vi "serial_AUCT_comp_p4.vi"() -> ()   [LabVIEW 2018]
uses:
  Controls created/Control 3.ctl
  Controls created/Control 4.ctl
  <vilib>/Instr/_visa.llb/VISA Configure Serial Port (Instr).vi
  <instrlib>/LeCroy Wave Series/Public/Data/Read Single Waveform.vi
  <vilib>/Utility/file.llb/Read Delimited Spreadsheet (DBL).vi
  <vilib>/Utility/file.llb/Write Delimited Spreadsheet (DBL).vi
  <instrlib>/Siglent SDG X Series/Siglent SDG X Series.lvlib
  <instrlib>/LeCroy Wave Series/LeCroy Wave Series.lvlib
panel:
  out "relative seconds 2":dbl format="%_19f"
  out "relative seconds":dbl
  out "Array":dbl[][](array[numeric])
  in  "Tab Control":T1(tab)
  in  "Scanning Distance(in mm)":i32=26
  in  "Experiment Dir":path=path "E:/Ankur/Labview/Automation/Data"
  in  "Exp_name":string="Test1"
  out "Exp_dir out dir":path
  out "Proc_data out dir":path
  out "Dis_step":dbl
  in  "Trend":dbl
  in  "N_packets":dbl=7.0
  out "Sinogram":dbl[][](graph)
  out "Reconstruction":dbl[][](graph)
  in  "VISA resource":refnum<visa-resource-name>="COM5"
  in  "NR":i16=10
  in  "Set Speed (Steps/s)":i16=900 min=0 max=3000 step=50
  in  "Baud Rate":u32=9600
  out "Iteration #":i32
  in  "NT":i16=10
  out "Error":errorcluster
  in  "Arbitray Movement":bool
  out "stop motion":bool
  in  "MOTION":bool
  in  "?":i8(slide) step=2 scale=0.0..2.0
  in  "OK Button":bool
  out "# NT":i32
  in  "ms to wait(Translation)":u32=100
  in  "milliseconds to wait":u32=100
  in  "ms to wait(Rotation)":u32=100
  out "Code Part Time":dbl[](array[numeric])
  out "gr_time":dbl
  in  "VISA Refnum in":refnum<visa-resource-name>="USB0::0xF4EC::0xEE38::SDG2XCAD2R3765::INSTR"
  in  "Channel (1:Channel 1)":i32(ring)=1 items=["Channel 1"=1, "Channel 2"=2]
  in  "Enable Output (T: Enable)":bool=TRUE
  in  "Amplitude (1.0 Vpp)":dbl=20.0 format="%#.3f"
  in  "Frequency (1000 Hz)":T2=1500000.0 format="%#.6g"
  in  "DC Offset (0.00 V) in":dbl
  in  "Waveform Function (0: Sine) in":u16(ring) items=["Sine", "Square", "Ramp", "DC", "Pulse", "Arb"]
  in  "Phase (0.0 degrees)":dbl=0.002 min=-360.0 max=360.0 format="%#.1g"
  in  "Fall (20 ns)":dbl=8.4e-09 format="%#.3g"
  in  "Duty (20%)":dbl=4.32 min=0.0001 max=100.0 format="%.4g"
  in  "Delay (0.00 s)":dbl min=-1000000.0 max=1000000.0
  in  "Rise (20 ns)":dbl=1.04e-08 format="%#.3g"
  in  "True To \ngenerate\n pulse":T3=TRUE
  out "VISA resource name out":refnum<visa-resource-name>
  out "error out":errorcluster
  out "Output Filename":path
  out "error out 2":errorcluster
  in  "format string":string="Channel: %g \nWavetype: %g \nAMP: %gV\nFreq: %gHz \nRiseTime: %gs \nFallTime: %gs \nDutyCycle: %g"
  out "Oscilloscope\n Runnning":bool
  in  "stop":bool
  out "Waveform Data":waveform(dbl)(graph)
  in  "Source (0: Channel 1)":u16(ring) items=["Channel 1", "Channel 2", "Channel 3", "Channel 4", "Memory 1", "Memory 2", "Memory 3", "Memory 4", "Function 1", "Function 2", "Function 3", "Function 4", "Function 5", "Function 6", "Function 7", "Function 8"]
  in  "Perform Auto Setup?":bool
  in  "Save Files in Directory (In Oscilloscope)":string="D:\\Automation\\Data"
  in  "Filename":string="Title"
  out "Saved filename":string
  out "Error Dsocom":errorcluster
  in  "VISA resource name":refnum<visa-resource-name>="USB0::0x05FF::0x1023::3517N53447::INSTR"
  in  "Reset Scope?":bool
  out "VISA DSO":refnum<visa-resource-name>
  # "For Rotational motion"
  # "For Translational Motion"
  # "For Translational motion"
  # "OFF"
  # "ON"
  # "Instr conn"
  # "Scan. loop"
  # "All Comb"
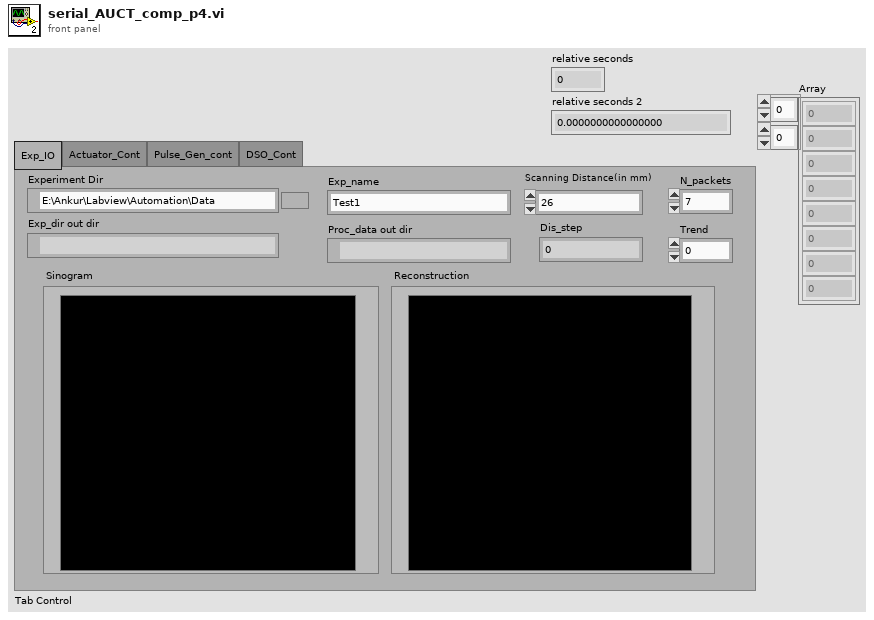
[diagram p1: front panel]
types:
  T1 = enum32{"Exp_IO", "Actuator_Cont", "Pulse_Gen_cont", "DSO_Cont"}
  T2 = typedef "Control 3.ctl" = dbl
  T3 = typedef "Control 4.ctl" = bool
  T4 = enum16{"open", "replace", "create", "open or create", "replace or create", "replace or create with confirmation"}
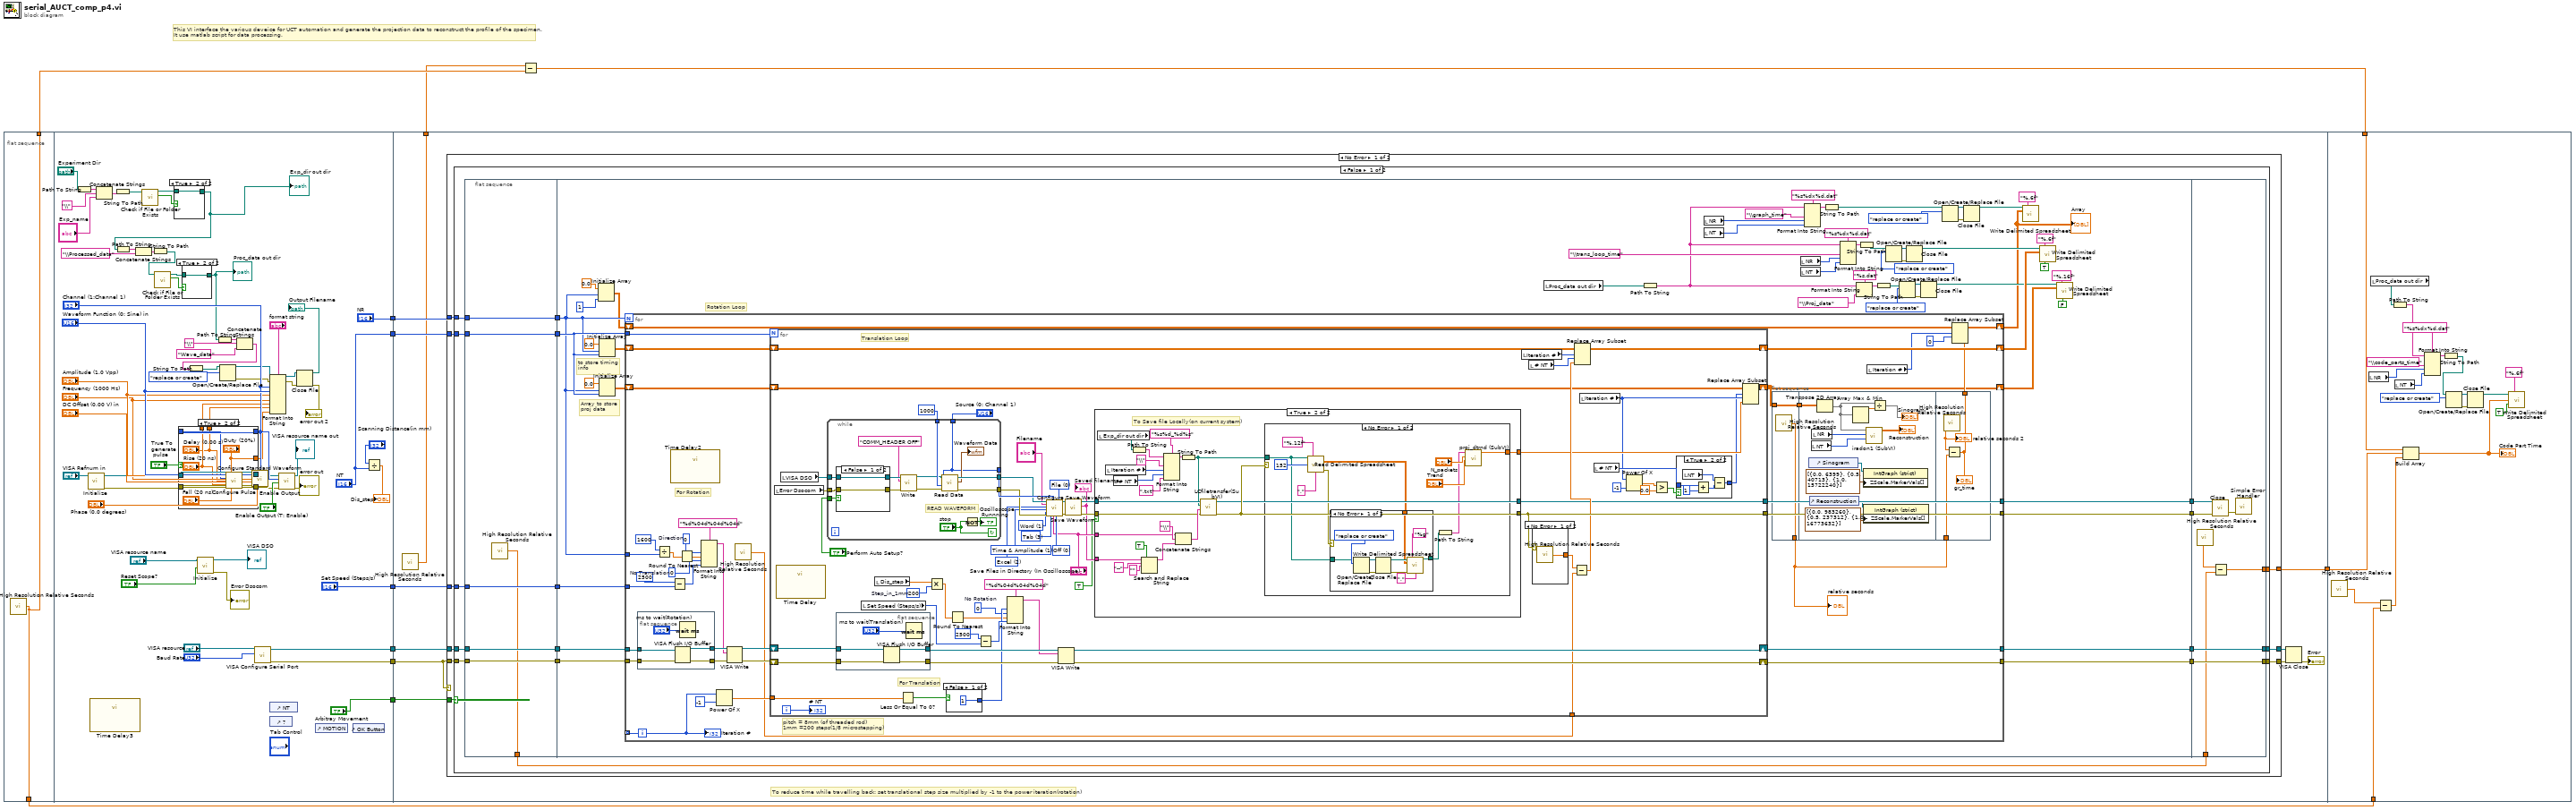
[diagram p0: block diagram]
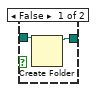
[diagram p2: hidden frame]
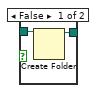
[diagram p3: hidden frame]
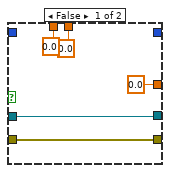
[diagram p4: hidden frame]
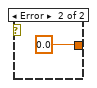
[diagram p6: hidden frame]
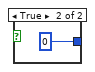
[diagram p7: hidden frame]
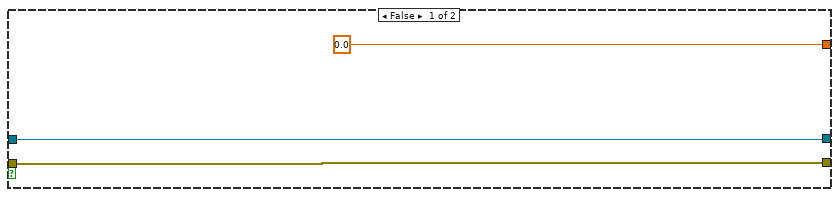
[diagram p8: hidden frame]
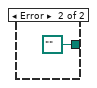
[diagram p9: hidden frame]
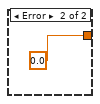
[diagram p10: hidden frame]
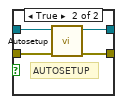
[diagram p11: hidden frame]
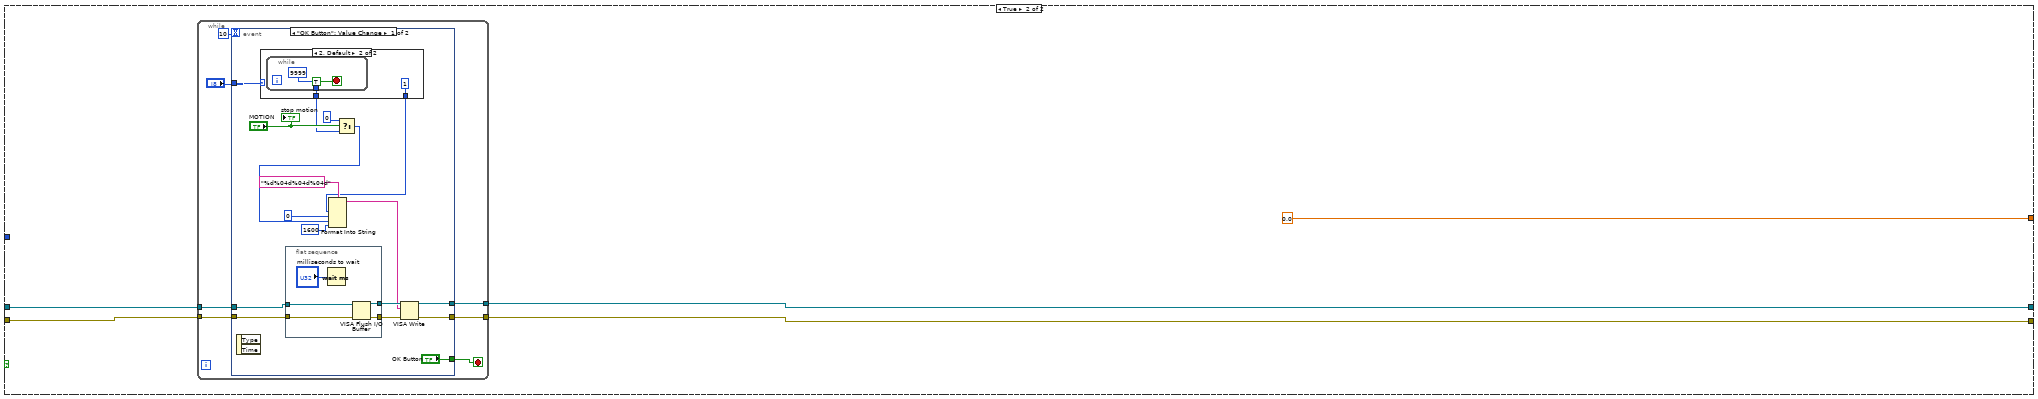
[diagram p12: hidden frame]
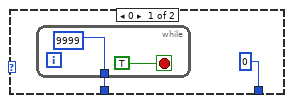
[diagram p13: hidden frame]
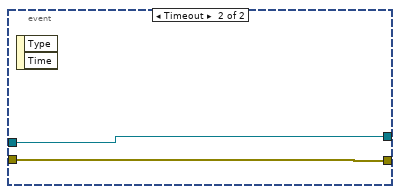
[diagram p14: hidden frame]
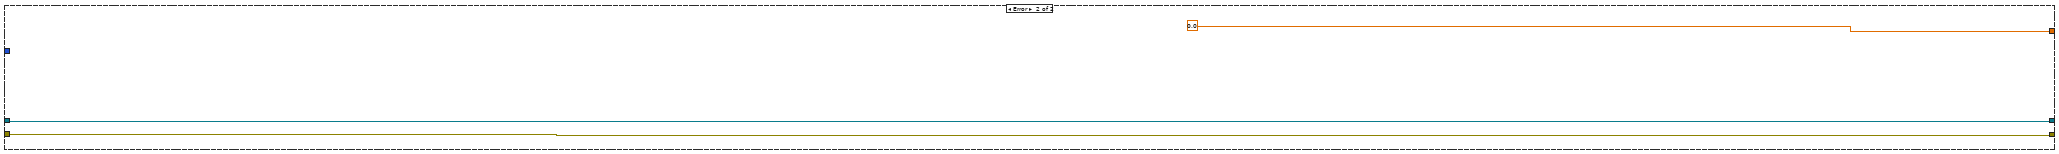
[diagram p15: hidden frame]
diagram:
  # "This VI interface the various deveice for UCT automation and generate the projection data to reconstruct the profile of the specimen.\nIt use matlab script for data processing."
  n1 = flat-sequence {
    tunnel: [w12] -> w3
    tunnel: [w12] -> w2
    tunnel: ["NT"] -> w11
    tunnel: [w41] -> w10
    tunnel: [w40] -> w9
    tunnel: ["Arbitray Movement"] -> w8
    tunnel: ["Set Speed (Steps/s)"] -> w7
    tunnel: ["NR"] -> w6
    tunnel: w11 -> [w103]
    tunnel: w10 -> [w102]
    tunnel: w9 -> [w101]
    tunnel: w8 -> [w100]
    tunnel: w7 -> [w99]
    tunnel: w6 -> [w98]
    tunnel: [w97] -> w4
    tunnel: [w96] -> w1
    tunnel: w5 -> [w471]
    tunnel: w4 -> [w470]
    tunnel: w3 -> [w469]
    frame #0 {
      n2 = call <vilib>:"High Resolution Relative Seconds.vi"() -> ("relative seconds"=w12:dbl)
    }
    frame #1 {
      n3 = Path To String(path="Experiment Dir") -> (string=w34:string)
      n4 = call <instrlib>:"Initialize.vi"("VISA resource name"="VISA Refnum in") -> ("error out"=w48:errorcluster, "VISA resource name out"=w47:refnum<visa-resource-name>)  [unwired: 9 in]
      n5 = call "Time Delay3"() -> ()  [unwired: 11 in, 1 out]
      n6 = Concatenate Strings(w34, "\\" ("string"), "Exp_name") -> (w32:string)
      n7 = String To Path(string=w32) -> (path=w28:path)
      n8 = call <vilib>:"Check if File or Folder Exists.vi"("path"=w28) -> ("file or folder exists?"=w27:bool, "dup path"=w26:path)  [unwired: 8 in, 1 out]
      n9 = case shown="True" w27 {
        tunnel: w26 -> [w80 w81]
        tunnel: [w79 w81] -> w22
        frame False {
          n10 = Create Folder(path (use dialog)=w80) -> (created path=w79:path)  [unwired: 2 in, 2 out]
        }
        frame True {
        }
      }
      "Exp_dir out dir" <- w22
      n11 = Path To String(path=w22) -> (string=w36:string)
      n12 = Concatenate Strings(w36, "\\Processed_data" ("string")) -> (w35:string)
      n13 = String To Path(string=w35) -> (path=w23:path)
      n14 = call <vilib>:"Check if File or Folder Exists.vi"("path"=w23) -> ("file or folder exists?"=w25:bool, "dup path"=w24:path)  [unwired: 8 in, 1 out]
      n15 = case shown="True" w25 {
        tunnel: [w77 w78] -> w19
        tunnel: w24 -> [w76 w78]
        frame False {
          n16 = Create Folder(path (use dialog)=w76) -> (created path=w77:path)  [unwired: 2 in, 2 out]
        }
        frame True {
        }
      }
      "Proc_data out dir" <- w19
      n17 = call <instrlib>:"Initialize.vi"("Reset? (T: Yes)"="Reset Scope?", "VISA resource name"="VISA resource name") -> ("error out"=→"Error Dsocom":errorcluster, "VISA resource name out"=→"VISA DSO":refnum<visa-resource-name>)  [unwired: 8 in]
      n18 = Path To String(path=w19) -> (string=w20:string)
      n19 = Concatenate Strings(w20, "\\" ("string"), "Wave_data" ("Filename")) -> (w16:string)
      n20 = String To Path(string=w16) -> (path=w15:path)
      n21 = Open/Create/Replace File(file path (use dialog)=w15, operation (0:open)=T4."replace or create") -> (refnum out=w21:refnum<file>, error out=w13:errorcluster)  [unwired: 4 in, 1 out]
      n22 = call <instrlib>:"Configure Standard Waveform.vi"("VISA resource name"=w47, "Waveform Function (0: Sine)"="Waveform Function (0: Sine) in", "Channel (1:Channel 1)"="Channel (1:Channel 1)", "Amplitude (1.0 Vpp)"="Amplitude (1.0 Vpp)", "Frequency (1000 Hz)"="Frequency (1000 Hz)", "DC Offset (0.00 V)"="DC Offset (0.00 V) in", "error in (no error)"=w48, "Phase (0.0 degrees)"="Phase (0.0 degrees)") -> ("VISA resource name out"=w52:refnum<visa-resource-name>, "error out"=w49:errorcluster)  [unwired: 6 in]
      n23 = case shown="True" "True To \ngenerate\n pulse" {
        tunnel: [w86 w94] -> w43
        tunnel: [w85 w93] -> w44
        tunnel: w52 -> [w86 w92]
        tunnel: w49 -> [w85 w91]
        tunnel: "Channel (1:Channel 1)" -> [_ w90]
        tunnel: "Channel (1:Channel 1)" -> [_ _]
        tunnel: [0.0 ("Duty (20%)") "Duty (20%)"] -> w56
        tunnel: [0.0 ("Rise (20 ns)") "Rise (20 ns)"] -> w64
        tunnel: [0.0 ("Delay (0.00 s)") "Delay (0.00 s)"] -> w65
        frame False {
        }
        frame True {
          n24 = call <instrlib>:"Configure Pulse.vi"("VISA resource name"=w92, "Duty (20%)"="Duty (20%)", "Channel (1:Channel 1)"=w90, "Delay (0.00 s)"="Delay (0.00 s)", "Rise (20 ns)"="Rise (20 ns)", "error in (no error)"=w91, "Fall (20 ns)"="Fall (20 ns)") -> ("VISA resource name out"=w94:refnum<visa-resource-name>, "error out"=w93:errorcluster)  [unwired: 7 in]
        }
      }
      n25 = call-poly "VISA Configure Serial Port"("VISA resource name"="VISA resource", "baud rate (9600)"="Baud Rate") -> ("VISA resource name out"=w41:refnum<visa-resource-name>, "error out"=w40:errorcluster)  [unwired: 12 in]
      n26 = Format Into String(format string="format string", initial string=w21, error in=w13, "Channel (1:Channel 1)", "Waveform Function (0: Sine) in", "Amplitude (1.0 Vpp)", "Frequency (1000 Hz)", w64, w65, w56) -> (resulting string=w57:refnum<file>, error out=w60:errorcluster)
      n27 = control-ref of="NT"() -> ()  [unwired: 1 out]
      n28 = control-ref of="?"() -> ()  [unwired: 1 out]
      n29 = call <instrlib>:"Enable Output.vi"("error in (no error)"=w44, "Enable Output (T: Enable)"="Enable Output (T: Enable)", "Channel (1:Channel 1)"="Channel (1:Channel 1)", "VISA resource name"=w43) -> ("error out"=→"error out":errorcluster, "VISA resource name out"=→"VISA resource name out":refnum<visa-resource-name>)  [unwired: 6 in]
      n30 = Close File(refnum=w57, error in=w60) -> (path=→"Output Filename":path, error out=→"error out 2":errorcluster)
      n31 = control-ref of="MOTION"() -> ()  [unwired: 1 out]
      n32 = control-ref of="OK Button"() -> ()  [unwired: 1 out]
      n33 = Divide(x="Scanning Distance(in mm)", y="NT") -> (x/y=→"Dis_step":dbl)
    }
    frame #2 {
      # "To reduce time while travelling back: set translational step size multiplied by -1 to the power iteration(rotation)"
      n34 = call <vilib>:"High Resolution Relative Seconds.vi"() -> ("relative seconds"=w96:dbl)
      n35 = case shown="No Error" w101 {
        tunnel: [w108 w451] -> w106
        tunnel: w98 -> [w115 _]
        tunnel: w99 -> [w114 _]
        tunnel: w100 -> [w113 _]
        tunnel: w101 -> [w112 w451]
        tunnel: w102 -> [w111 w450]
        tunnel: w103 -> [w110 _]
        tunnel: [w109 w450] -> w104
        tunnel: [w107 0.0] -> w97
        frame No Error {
          n36 = case shown="False" w113 {
            tunnel: w115 -> [w130 _]
            tunnel: w114 -> [w133 _]
            tunnel: w112 -> [w132 w409]
            tunnel: w111 -> [w131 w408]
            tunnel: w110 -> [w129 _]
            tunnel: [w128 w407] -> w109
            tunnel: [w118 w406] -> w108
            tunnel: [w117 0.0] -> w107
            frame False {
              n37 = flat-sequence {
                tunnel: w129 -> [w135]
                tunnel: w130 -> [w136]
                tunnel: w131 -> [w137]
                tunnel: w132 -> [w138]
                tunnel: w133 -> [w139]
                tunnel: [w139] -> w125
                tunnel: [w138] -> w124
                tunnel: [w137] -> w123
                tunnel: [w136] -> w122
                tunnel: [w135] -> w121
                tunnel: [w134] -> w116
                tunnel: [w190] -> w127
                tunnel: [w189] -> w126
                tunnel: w125 -> [w193]
                tunnel: w124 -> [w192]
                tunnel: w123 -> [w191]
                tunnel: w122 -> [w143]
                tunnel: w121 -> [w170]
                tunnel: [w188] -> w120
                tunnel: [w187] -> w119
                tunnel: [w404] -> w128
                tunnel: w127 -> [w404]
                tunnel: w126 -> [w400]
                tunnel: w120 -> [w402]
                tunnel: w119 -> [w401]
                tunnel: [w400] -> w118
                tunnel: [w398] -> w117
                tunnel: w116 -> [w397]
                frame #0 {
                  n38 = call <vilib>:"High Resolution Relative Seconds.vi"() -> ("relative seconds"=w134:dbl)
                }
                frame #1 {
                  # "to store timing\ninfo"
                  # "Array to store \nproj data"
                  # "Rotation Loop"
                  n39 = Initialize Array(0.0 ("element"), w143, 1 ("dimension size")) -> (w142:dbl[][])
                  n40 = Initialize Array(0.0, w143, w170) -> (w173:dbl[][])
                  n41 = Initialize Array(0.0, w143, w170) -> (w169:dbl[][])
                  n42 = for {
                    N: w143 -> [_]
                    tunnel: [w227] -> w189
                    tunnel: [w228] -> w190
                    tunnel: w193 -> [w208]
                    tunnel: [w230] -> _ mode=indexing
                    tunnel: w192 -> [w221]
                    tunnel: w191 -> [w222]
                    tunnel: w143 -> [w214]
                    tunnel: w170 -> [w210]
                    tunnel: [w207] -> w188
                    tunnel: [w206] -> w187
                    shift-right: [w203] -> w172
                    shift-left: w173 -> [w204]
                    shift-right: [w194] -> w157
                    shift-left: w169 -> [w202]
                    shift-right: [w199] -> w141
                    shift-left: w142 -> [w200]
                    i -> [w230]
                    w218 = 0  # No Translation
                    w216 = 0  # Direction
                    # "pitch = 8mm (of threaded rod)\n1mm =200 steps(1/8 microstepping)"
                    # "For Rotation"
                    n43 = flat-sequence {
                      tunnel: [w251] -> w225
                      tunnel: [w250] -> w226
                      tunnel: w222 -> [w248]
                      tunnel: w221 -> [w247]
                      frame #0 {
                        n44 = VISA Flush I/O Buffer(VISA resource name=w248, error in (no error)=w247) -> (VISA resource name out=w251:refnum<visa-resource-name>, error out=w250:errorcluster)  [unwired: 1 in]
                        n45 = Wait (ms)(milliseconds to wait="ms to wait(Rotation)") -> ()  [unwired: 1 out]
                      }
                    }
                    n46 = Divide(x=i16 1600, y=w214) -> (x/y=w213:dbl)
                    n47 = call "Time Delay2"() -> ()  [unwired: 11 in, 1 out]
                    n48 = Subtract(x=i16 2500 ("y"), y=w208) -> (x-y=w217:i16)
                    n49 = Round To Nearest(number=w213) -> (nearest integer value=w212:dbl)
                    n50 = Format Into String(format string="%d%04d%04d%04d", w216, w212, w218, w217) -> (resulting string=w220:string)  [unwired: 2 in, 1 out]
                    n51 = Power Of X(1:-1 ("x"), 2:w230) -> (0:w211:dbl)
                    n52 = VISA Write(VISA resource name=w225, write buffer=w220, error in (no error)=w226) -> (VISA resource name out=w223:refnum<visa-resource-name>, error out=w224:errorcluster)  [unwired: 1 out]
                    n53 = call <vilib>:"High Resolution Relative Seconds.vi"() -> ("relative seconds"=w205:dbl)
                    n54 = for {
                      N: w210 -> [_]
                      shift-right: [w281] -> w228
                      shift-left: w223 -> [w291]
                      shift-right: [w280] -> w227
                      shift-left: w224 -> [w290]
                      tunnel: w211 -> [w284]
                      tunnel: [w272] -> w207
                      tunnel: [w260] -> w206
                      tunnel: w205 -> [w270]
                      shift-right: [w268] -> w203
                      shift-left: w204 -> [w265]
                      shift-right: [w252] -> w194
                      shift-left: w202 -> [w264]
                      i -> [w312]
                      w276 = 200  # Step_in_1mm
                      w279 = 0  # No Rotation
                      w302 = u16 3 items=["Comma", "Space", "Semicolon", "Tab"] ("Delimiter (  0:Comma)")
                      w301 = u16 0 items=["Off", "Wrap", "Fill"] ("Auto Save (0:Off")
                      w303 = u16 1 items=["Byte", "Word", "Auto"] ("BinarySubFormat (1: Word)")
                      w304 = u16 1 items=["Amplitude Only", "Time & Amplitude", "With Header"] ("SubFormat (1: Time & Amplitude)")
                      w305 = u16 2 items=["Binary", "ASCII", "Excel", "MATLAB", "MathCad", "WaveML"] ("Format (0: Binary)")
                      w300 = u16 0 items=["File", "M1", "M2", "M3", "M4"] ("Destination (0:File)")
                      # "Translation Loop"
                      # "For Translation"
                      n55 = local read "Error Dsocom"() -> (w261:errorcluster)
                      n56 = call "Time Delay"() -> ()  [unwired: 11 in, 1 out]
                      n57 = local read "VISA DSO"() -> (w262:refnum<visa-resource-name>)
                      n58 = while {
                        tunnel: [w390] -> w310
                        tunnel: [w389] -> w309
                        tunnel: "Perform Auto Setup?" -> [w388]
                        tunnel: "Source (0: Channel 1)" -> [w382]
                        tunnel: w262 -> [w387]
                        tunnel: u32 1000 ("Timeout (10000 ms)") -> [w386]
                        tunnel: [w382] -> w311
                        tunnel: w261 -> [w381]
                        stop <- "stop" continue-if-true
                        # "READ WAVEFORM"
                        n59 = case shown="False" w388 {
                          tunnel: w381 -> [w391 w396]
                          tunnel: w387 -> [w392 w395]
                          tunnel: [w392 w394] -> w378
                          tunnel: [w391 w393] -> w377
                          frame False {
                          }
                          frame True {
                            # "AUTOSETUP"
                            n60 = call <instrlib>:"Autosetup.vi"("error in (no error)"=w396, "VISA resource name"=w395) -> ("error out"=w393:errorcluster, "VISA resource name out"=w394:refnum<visa-resource-name>)  [unwired: 8 in]
                          }
                        }
                        n61 = call <instrlib>:"Write.vi"("error in (no error)"=w377, "Write Buffer"="COMM_HEADER OFF", "VISA resource name"=w378) -> ("error out"=w379:errorcluster, "VISA resource name out"=w380:refnum<visa-resource-name>)  [unwired: 7 in]
                        n62 = call-poly <instrlib>:"Read Data.vi"("error in (no error)"=w379, "Timeout (10000 ms)"=w386, "Source (0: Channel 1)"=w382, "VISA resource name"=w380) -> ("error out"=w390:errorcluster, "Waveform Data"=→"Waveform Data":waveform(dbl), "VISA resource name out"=w389:refnum<visa-resource-name>)  [unwired: 5 in]
                        n63 = Not(x="stop") -> (.not. x?=→"Oscilloscope\n Runnning":bool)
                      }
                      n64 = flat-sequence {
                        tunnel: [w327] -> w289
                        tunnel: [w326] -> w288
                        tunnel: w291 -> [w324]
                        tunnel: w290 -> [w323]
                        frame #0 {
                          n65 = VISA Flush I/O Buffer(VISA resource name=w324, error in (no error)=w323) -> (VISA resource name out=w327:refnum<visa-resource-name>, error out=w326:errorcluster)  [unwired: 1 in]
                          n66 = Wait (ms)(milliseconds to wait="ms to wait(Translation)") -> ()  [unwired: 1 out]
                        }
                      }
                      n67 = local read "Set Speed (Steps/s)"() -> (w273:i16)
                      n68 = local read "Dis_step"() -> (w277:dbl)
                      n69 = Less Or Equal To 0?(x=w284) -> (x <= 0?=w283:bool)
                      n70 = Multiply(x=w277, y=w276) -> (x*y=w275:dbl)
                      n71 = case shown="False" w283 {
                        tunnel: [1 0] -> w282
                        frame False {
                        }
                        frame True {
                        }
                      }
                      n72 = Round To Nearest(number=w275) -> (nearest integer value=w278:dbl)
                      n73 = Subtract(x=i16 2500 ("y"), y=w273) -> (x-y=w287:i16)
                      n74 = Format Into String(format string="%d%04d%04d%04d", w282, w279, w278, w287) -> (resulting string=w285:string)  [unwired: 2 in, 1 out]
                      n75 = call <instrlib>:"Configure Save Waveform.vi"("VISA resource name"=w309, "Trace Title (Title)"="Filename", "Format (0: Binary)"=w305, "SubFormat (1: Time & Amplitude)"=w304, "BinarySubFormat (1: Word)"=w303, "error in (no error)"=w310, "Delimiter (  0:Comma)"=w302, "Source (0: Channel 1)"=w311, "Save Files in Directory (D:\\Waveforms)"="Save Files in Directory (In Oscilloscope)", "Auto Save (0:Off"=w301, "Destination (0:File)"=w300) -> ("VISA resource name out"=w299:refnum<visa-resource-name>, "error out"=w298:errorcluster)  [unwired: 7 in]
                      n76 = VISA Write(VISA resource name=w289, write buffer=w285, error in (no error)=w288) -> (VISA resource name out=w281:refnum<visa-resource-name>, error out=w280:errorcluster)  [unwired: 1 out]
                      n77 = call <instrlib>:"Save Waveform.vi"("error in (no error)"=w298, "VISA resource name"=w299) -> ("error out"=w296:errorcluster, "Saved filename"=w294:string, "VISA resource name out"=w295:refnum<visa-resource-name>)  [unwired: 7 in]
                      "Saved filename" <- w294
                      n78 = case shown="True" TRUE ("Save File locally") {
                        tunnel: [w329 w332] -> w272
                        tunnel: "Save Files in Directory (In Oscilloscope)" -> [_ w346]
                        tunnel: w296 -> [w329 w345]
                        tunnel: w295 -> [w330 w344]
                        tunnel: w294 -> [_ w343]
                        tunnel: [0.0 ("Real") w337] -> w263
                        tunnel: [w330 w331] -> w260
                        frame False {
                        }
                        frame True {
                          # "To Save file Locally(on current system)"
                          n79 = local read "Exp_dir out dir"() -> (w336:path)
                          n80 = local read "Iteration #"() -> (w334:i32)
                          n81 = local read "# NT"() -> (w333:i32)
                          n82 = Path To String(path=w336) -> (string=w347:string)
                          n83 = Search and Replace String(replace all?=TRUE ("replace all? (F)"), input string=w343, search string="--", replace string="" ("replace string (\"\")")) -> (result string=w342:string)  [unwired: 4 in, 3 out]
                          n84 = Format Into String(format string="%s%d_%d%s", initial string=w347, "\\" ("input 1"), w334, w333, ".txt" ("input 3")) -> (resulting string=w340:string)  [unwired: 1 in, 1 out]
                          n85 = Concatenate Strings(w346, "\\" ("string"), w342) -> (w350:string)
                          n86 = String To Path(string=w340) -> (path=w335:path)
                          n87 = call <userlib>:"LCfiletransfer(SubVI).vi"("error in (no error)"=w345, "Source Filename"=w350, "file path (use dialog)"=w335, "VISA Refnum in"=w344) -> ("error out"=w332:errorcluster, "VISA Refnum out"=w331:refnum<visa-resource-name>)  [unwired: 5 in, 1 out]
                          n88 = case shown="No Error" w332 {
                            tunnel: [w360 0.0 ("Real")] -> w337
                            tunnel: w335 -> [w356 _]
                            frame No Error {
                              n89 = call-poly <vilib>:"Read Delimited Spreadsheet.vi"("file path (dialog if empty)"=w356, "format (%.3f)"="%.12f", "start of read offset (chars.:0)"=152, "delimiter (\\t)"="," ("delimiter (\\t)")) -> ("all rows"=w357:dbl[][], "error out"=w355:errorcluster)  [unwired: 6 in, 4 out]
                              n90 = case shown="No Error" w355 {
                                tunnel: w357 -> [w367 _]
                                tunnel: w356 -> [w366 _]
                                tunnel: [w365 path "" ("new file path (Not A Path if cancelled)")] -> w354
                                frame No Error {
                                n91 = Open/Create/Replace File(file path (use dialog)=w366, operation (0:open)=T4."replace or create") -> (refnum out=w373:refnum<file>, error out=w372:errorcluster)  [unwired: 4 in, 1 out]
                                n92 = Close File(refnum=w373, error in=w372) -> (path=w371:path, error out=w370:errorcluster)
                                n93 = call-poly <vilib>:"Write Delimited Spreadsheet.vi"("file path (dialog if empty)"=w371, "format (%.3f)"="%g", "2D data"=w367, "error in (no error)"=w370, "delimiter (\\t)"="," ("delimiter (\\t)")) -> ("new file path (Not A Path if cancelled)"=w365:path)  [unwired: 9 in, 1 out]
                                }
                                frame Error {
                                }
                              }
                              n94 = Path To String(path=w354) -> (string=w353:string)
                              n95 = call "proj_dtrnd (SubVI).vi"("Trend"="Trend", "N_packets"="N_packets", "String"=w353) -> ("Real"=w360:dbl)  [unwired: 7 in, 1 out]
                            }
                            frame Error {
                            }
                          }
                        }
                      }
                      n96 = local read "Iteration #"() -> (w269:i32)
                      n97 = local read "# NT"() -> (w267:i32)
                      n98 = case shown="No Error" w272 {
                        tunnel: [w319 0.0] -> w271
                        frame No Error {
                          n99 = call <vilib>:"High Resolution Relative Seconds.vi"() -> ("relative seconds"=w319:dbl)
                        }
                        frame Error {
                        }
                      }
                      n100 = Subtract(x=w271, y=w270) -> (x-y=w266:dbl)
                      n101 = Replace Array Subset(array=w265, new element=w266, index (row)=w269, index (col)=w267) -> (w268:dbl[][])
                      n102 = local read "Iteration #"() -> (w254:i32)
                      n103 = local read "# NT"() -> (w255:i32)
                      n104 = Power Of X(1:-1 ("x"), 2:w254) -> (0:w258:dbl)
                      n105 = Greater?(x=w258, y=0.0) -> (0:w256:bool)
                      n106 = case shown="True" w256 {
                        tunnel: w255 -> [w313 w316]
                        tunnel: [w313 w317] -> w253
                        frame False {
                        }
                        frame True {
                          n107 = local read "NT"() -> (w318:i16)
                          n108 = Add(x=w316, y=1) -> (x+y=w314:i32)
                          n109 = Subtract(x=w318, y=w314) -> (x-y=w317:i32)
                        }
                      }
                      n110 = Replace Array Subset(array=w264, new element=w263, index (row)=w253, index (col)=w254) -> (w252:dbl[][])
                      "# NT" <- w312
                    }
                    n111 = flat-sequence {
                      tunnel: [w232] -> w196
                      tunnel: [w231] -> w195
                      tunnel: w194 -> [w231]
                      tunnel: w195 -> [w233]
                      tunnel: [w245] -> w198
                      tunnel: w196 -> [w244]
                      frame #0 {
                        n112 = call <vilib>:"High Resolution Relative Seconds.vi"() -> ("relative seconds"=w232:dbl)
                      }
                      frame #1 {
                        n113 = control-ref of="Sinogram"() -> (w237:refnum<vi>)
                        n114 = control-ref of="Reconstruction"() -> (w236:refnum<vi>)
                        n115 = local read "NT"() -> (w242:i16)
                        n116 = local read "NR"() -> (w243:i16)
                        n117 = Transpose 2D Array(2D array=w233) -> (transposed array=w239:dbl[][])
                        n118 = Array Max & Min(array=w239) -> (max value=w240:dbl)  [unwired: 3 out]
                        n119 = property on="Property Node" class="IntGraph (strict)"(reference=w237, "ZScale.MarkerVals[]"=cluster{dbl, u32}[] [{0.0, 6399}, {0.5, 40713}, {1.0, 15722240}] ("Z Scale.Marker Values[]")) -> ()  [unwired: 1 in, 2 out]
                        n120 = property on="Property Node" class="IntGraph (strict)"(reference=w236, "ZScale.MarkerVals[]"=cluster{dbl, u32}[] [{0.0, 983260}, {0.5, 237312}, {1.0, 16773632}] ("Z Scale.Marker Values[]")) -> ()  [unwired: 1 in, 2 out]
                        n121 = call "iradon1 (SubVI).vi"("N_det"=w242, "N_rot"=w243, "2-D Array of Real"=w239) -> ("x/y"=→"Reconstruction":dbl[][])  [unwired: 8 in]
                        n122 = Divide(x=w239, y=w240) -> (x/y=→"Sinogram":dbl[][])
                      }
                      frame #2 {
                        n123 = call <vilib>:"High Resolution Relative Seconds.vi"() -> ("relative seconds"=w246:dbl)
                        "relative seconds 2" <- w246
                        n124 = Subtract(x=w246, y=w244) -> (x-y=w245:dbl)
                        "gr_time" <- w245
                      }
                    }
                    n125 = local read "Iteration #"() -> (w201:i32)
                    n126 = Replace Array Subset(array=w200, new element=w198, index (row)=w201, index (col)=0 ("disabled index (col)")) -> (w199:dbl[][])
                    "Iteration #" <- w230
                    "relative seconds" <- w196
                  }
                  "Array" <- w141
                  n127 = local read "Proc_data out dir"() -> (w166:path)
                  n128 = Path To String(path=w166) -> (string=w140:string)
                  n129 = local read "NR"() -> (w148:i16)
                  n130 = local read "NT"() -> (w147:i16)
                  n131 = local read "NR"() -> (w181:i16)
                  n132 = local read "NT"() -> (w182:i16)
                  n133 = Format Into String(format string="%s%dx%d.dat", initial string=w140, "\\graph_time" ("input 1"), w148, w147) -> (resulting string=w152:string)  [unwired: 1 in, 1 out]
                  n134 = String To Path(string=w152) -> (path=w146:path)
                  n135 = Format Into String(format string="%s%dx%d.dat", initial string=w140, "\\trans_loop_time", w181, w182) -> (resulting string=w184:string)  [unwired: 1 in, 1 out]
                  n136 = Format Into String(format string="%s.dat", initial string=w140, "\\Proj_data") -> (resulting string=w168:string)  [unwired: 1 in, 1 out]
                  n137 = String To Path(string=w184) -> (path=w185:path)
                  n138 = String To Path(string=w168) -> (path=w159:path)
                  n139 = Open/Create/Replace File(file path (use dialog)=w185, operation (0:open)=T4."replace or create") -> (refnum out=w177:refnum<file>, error out=w178:errorcluster)  [unwired: 4 in, 1 out]
                  n140 = Open/Create/Replace File(file path (use dialog)=w159, operation (0:open)=T4."replace or create") -> (refnum out=w162:refnum<file>, error out=w163:errorcluster)  [unwired: 4 in, 1 out]
                  n141 = Close File(refnum=w177, error in=w178) -> (path=w176:path)  [unwired: 1 out]
                  n142 = Close File(refnum=w162, error in=w163) -> (path=w161:path)  [unwired: 1 out]
                  n143 = Open/Create/Replace File(file path (use dialog)=w146, operation (0:open)=T4."replace or create") -> (refnum out=w154:refnum<file>, error out=w155:errorcluster)  [unwired: 4 in, 1 out]
                  n144 = Close File(refnum=w154, error in=w155) -> (path=w153:path)  [unwired: 1 out]
                  n145 = call-poly <vilib>:"Write Delimited Spreadsheet.vi"("file path (dialog if empty)"=w153, "format (%.3f)"="%.6f", "2D data"=w141) -> ()  [unwired: 11 in, 2 out]
                  n146 = call-poly <vilib>:"Write Delimited Spreadsheet.vi"("file path (dialog if empty)"=w176, "format (%.3f)"="%.6f", "2D data"=w172, "transpose? (no:F)"=TRUE) -> ()  [unwired: 10 in, 2 out]
                  n147 = call-poly <vilib>:"Write Delimited Spreadsheet.vi"("file path (dialog if empty)"=w161, "format (%.3f)"="%.16f", "2D data"=w157, "transpose? (no:F)"=FALSE) -> ()  [unwired: 10 in, 2 out]
                }
                frame #2 {
                  n148 = call <vilib>:"High Resolution Relative Seconds.vi"() -> ("relative seconds"=w399:dbl)
                  n149 = call <instrlib>:"Close.vi"("error in (no error)"=w402, "VISA resource name"=w401) -> ("error out"=w403:errorcluster)  [unwired: 9 in]
                  n150 = Subtract(x=w399, y=w397) -> (x-y=w398:dbl)
                  n151 = call <vilib>:"Simple Error Handler.vi"("error in (no error)"=w403) -> ()  [unwired: 4 in, 5 out]
                }
              }
            }
            frame True {
              n152 = while {
                tunnel: w409 -> [w414]
                tunnel: w408 -> [w413]
                tunnel: [w411] -> w407
                tunnel: [w412] -> w406
                stop <- w410 stop-if-true
                n153 = event shown="[0] \"OK Button\": Value Change" {
                  selector: _ -> [_ _]
                  dyn-events: _ -> [_ _]
                  timeout: 10 -> [_ _]
                  tunnel: "?" -> [w432 _]
                  tunnel: w414 -> [w422 w447]
                  tunnel: w413 -> [w423 w448]
                  tunnel: [w420 w447] -> w412
                  tunnel: [w421 w448] -> w411
                  tunnel: ["OK Button" _] -> w410
                  event "OK Button": Value Change {
                    n154 = event-data() -> ()  [unwired: 1 in, 2 out]
                    n155 = case shown="2, Default" w432 {
                      tunnel: [w440 w444] -> w430
                      tunnel: [0 ("input 1") 1 ("input 1")] -> w418
                      frame 0 {
                        n156 = while {
                          tunnel: [i16 9999 ("# of Steps to Move")] -> w440
                          stop <- TRUE ("Stop Reverse movement") stop-if-true
                        }
                      }
                      frame 2, Default {
                        n157 = while {
                          tunnel: [i16 9999 ("# of Steps to Move")] -> w444
                          stop <- TRUE ("Stop Forward movement") stop-if-true
                        }
                      }
                    }
                    n158 = flat-sequence {
                      tunnel: [w438] -> w429
                      tunnel: [w437] -> w428
                      tunnel: w423 -> [w435]
                      tunnel: w422 -> [w434]
                      frame #0 {
                        n159 = Wait (ms)(milliseconds to wait="milliseconds to wait") -> ()  [unwired: 1 out]
                        n160 = VISA Flush I/O Buffer(VISA resource name=w435, error in (no error)=w434) -> (VISA resource name out=w438:refnum<visa-resource-name>, error out=w437:errorcluster)  [unwired: 1 in]
                      }
                    }
                    n161 = Select(t=0, s="MOTION", f=w430) -> (s? t:f=w419:i32)
                    n162 = Format Into String(format string="%d%04d%04d%04d", w418, 0 ("input 2"), w419, 1600 ("input 4")) -> (resulting string=w426:string)  [unwired: 2 in, 1 out]
                    n163 = VISA Write(VISA resource name=w429, write buffer=w426, error in (no error)=w428) -> (VISA resource name out=w421:refnum<visa-resource-name>, error out=w420:errorcluster)  [unwired: 1 out]
                    "stop motion" <- "MOTION"
                  }
                  event Timeout {
                    n164 = event-data() -> ()  [unwired: 1 in, 2 out]
                  }
                }
              }
            }
          }
        }
        frame Error {
        }
      }
      n165 = VISA Close(VISA resource name=w104, error in (no error)=w106) -> (error out=→"Error":errorcluster)
    }
    frame #3 {
      n166 = call <vilib>:"High Resolution Relative Seconds.vi"() -> ("relative seconds"=w468:dbl)
      n167 = local read "NR"() -> (w457:i16)
      n168 = local read "Proc_data out dir"() -> (w454:path)
      n169 = Subtract(x=w468, y=w469) -> (x-y=w452:dbl)
      n170 = Path To String(path=w454) -> (string=w453:string)
      n171 = local read "NT"() -> (w456:i16)
      n172 = Build Array(w471, w470, w452) -> (w458:dbl[])
      "Code Part Time" <- w458
      n173 = Format Into String(format string="%s%dx%d.dat", initial string=w453, "\\code_parts_time", w457, w456) -> (resulting string=w460:string)  [unwired: 1 in, 1 out]
      n174 = String To Path(string=w460) -> (path=w459:path)
      n175 = Open/Create/Replace File(file path (use dialog)=w459, operation (0:open)=T4."replace or create") -> (refnum out=w466:refnum<file>, error out=w467:errorcluster)  [unwired: 4 in, 1 out]
      n176 = Close File(refnum=w466, error in=w467) -> (path=w463:path)  [unwired: 1 out]
      n177 = call-poly <vilib>:"Write Delimited Spreadsheet.vi"("file path (dialog if empty)"=w463, "format (%.3f)"="%.6f", "1D data"=w458, "transpose? (no:F)"=TRUE) -> ()  [unwired: 10 in, 2 out]
    }
  }
  n178 = Subtract(x=w1, y=w2) -> (x-y=w5:dbl)
